vi "CODMn流程质控自动启动.vi"(0 "参数":T1={"是否启用仪器"=FALSE, "CODMn"={"启动测量模式"={"测量模式"=enum."水样测量"}, "确定按钮"=TRUE}, "启动模块"={"氨氮"=FALSE, "总磷"=FALSE, "总氮"=FALSE, "COD"=FALSE}, "常规启动"=FALSE, "直接启动"=FALSE}, 1 "CODMn量程切换":enum32{"H", "L", "AUTO"}(ring)=enum."AUTO") -> ()   [LabVIEW 2016, in "质控单元.lvlib"]
uses:
  PLC/PLC.lvlib
panel:
  out "枚举 2":enum16{"初始化", "采配水启动", "等待", "配水", "排水", "结束"}(ring)
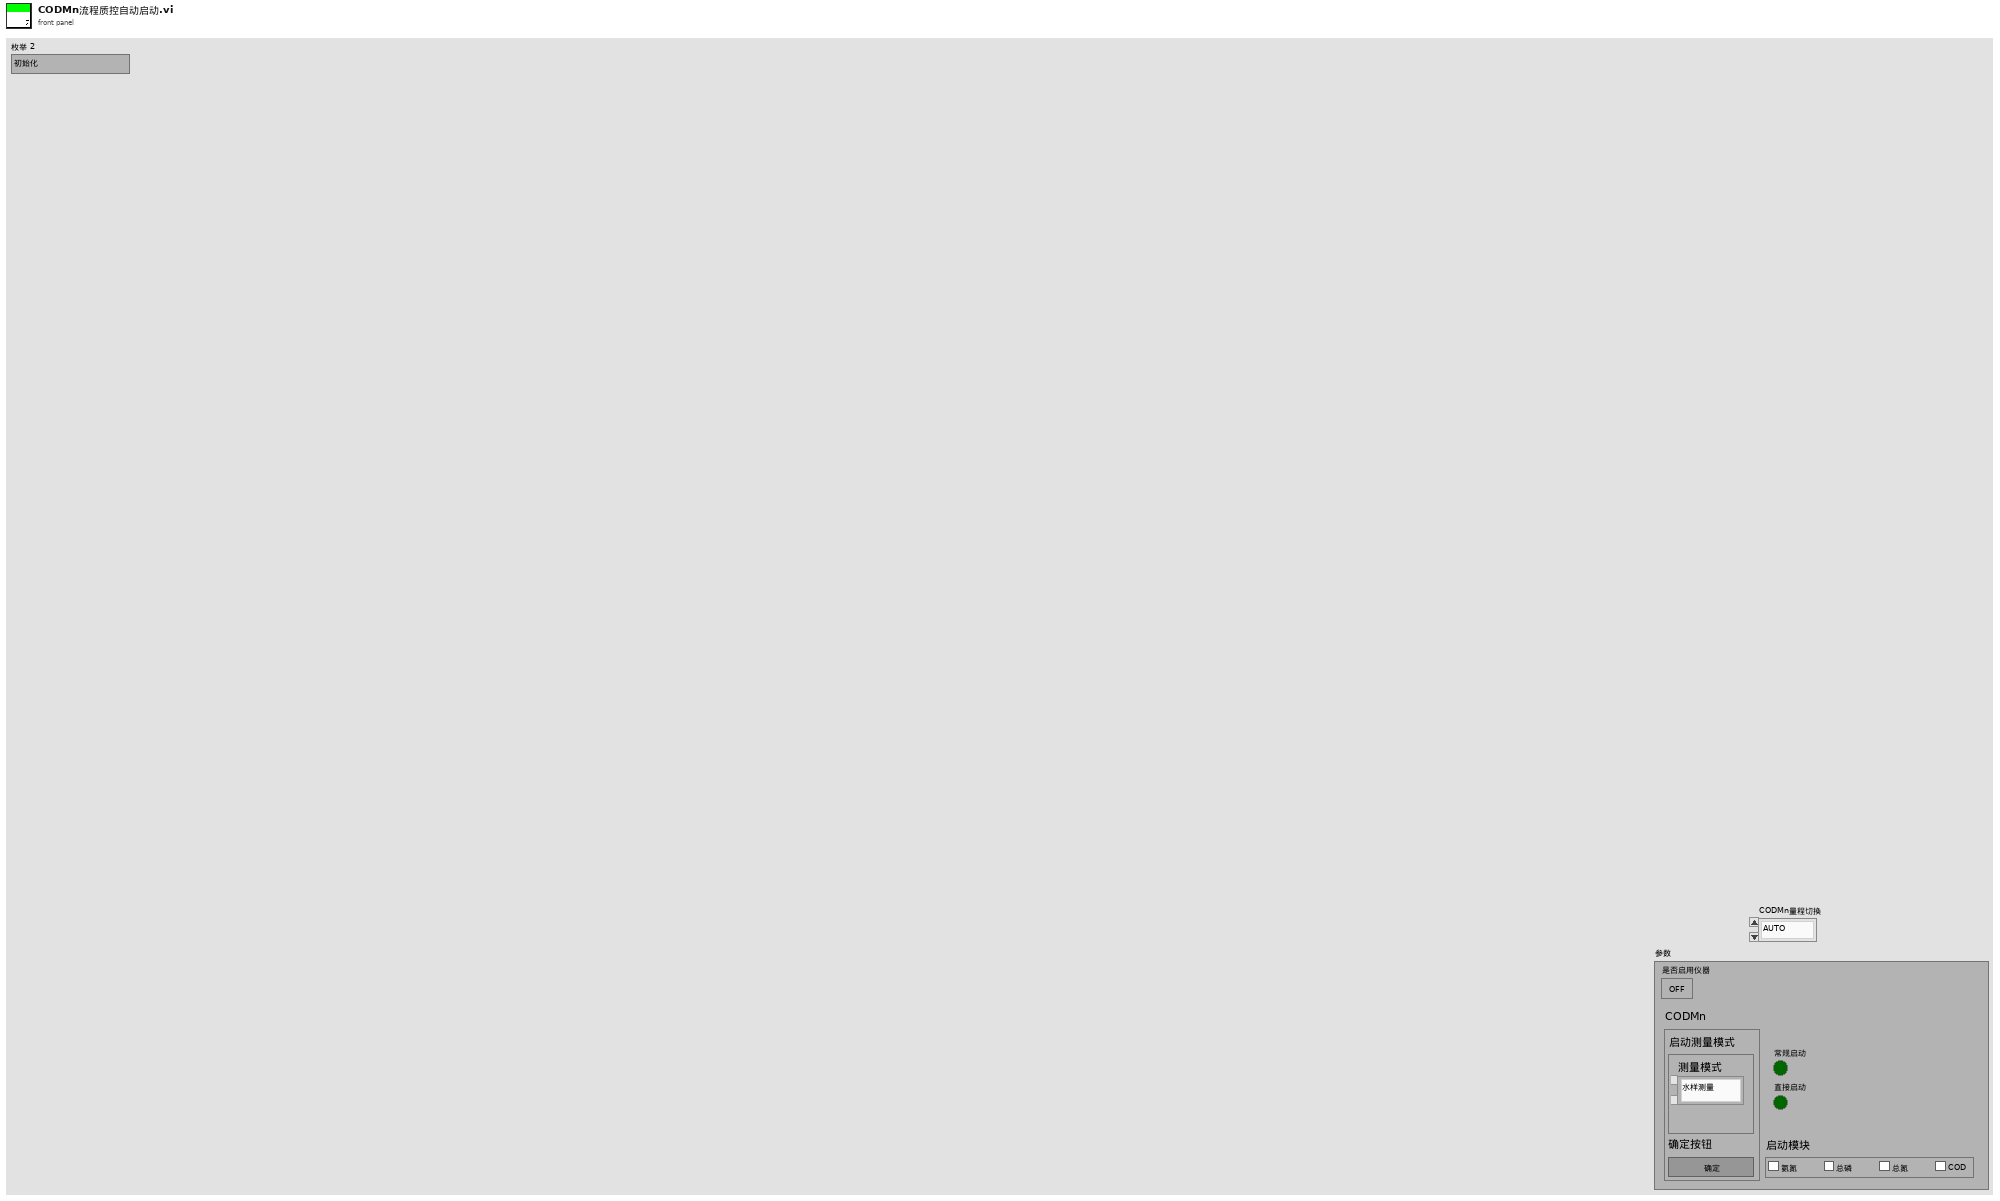
[diagram p1: front panel]
types:
  T1 = cluster{"是否启用仪器":bool, "CODMn":cluster{"启动测量模式":cluster{"测量模式":enum16{"水样测量", "标样核查", "加标回收", "平行样", "校零", "校标"}}, "确定按钮":bool}, "启动模块":cluster{"氨氮":bool, "总磷":bool, "总氮":bool, "COD":bool}, "常规启动":bool, "直接启动":bool}
  T2 = cluster{"R0":i16, "R1":i16, "R2":i16, "R3":i16, "R4":i16, "R5":i16, "R6":i16, "R7":i16, "R8":i16, "R9":i16, "R10":i16, "R11":i16, "R12":i16, "R13":i16, "R14":i16, "R15":i16, "R16":i16, "R17":i16, "R18":i16, "R19":i16, "R20":i16, "R21":i16, "R22":i16, "R23":i16, "R24":i16, "R25":i16, "R26":i16, "R27":i16, "R28":i16, "R29":i16, "R30":i16, "R31":i16, "R32":i16, "R33":i16, "R34":i16, "R35":i16, "R36":i16, "R37":i16, "R38":i16, "R39":i16, "R40":i16, "R41":i16, "R42":i16, "R43":i16, "R44":i16, "R45":i16, "R46":i16, "R47":i16, "R48":i16, "R49":i16, "R50":i16, "R51":i16, "R52":i16, "R53":i16, "R54":i16, "R55":i16, "R56":i16}
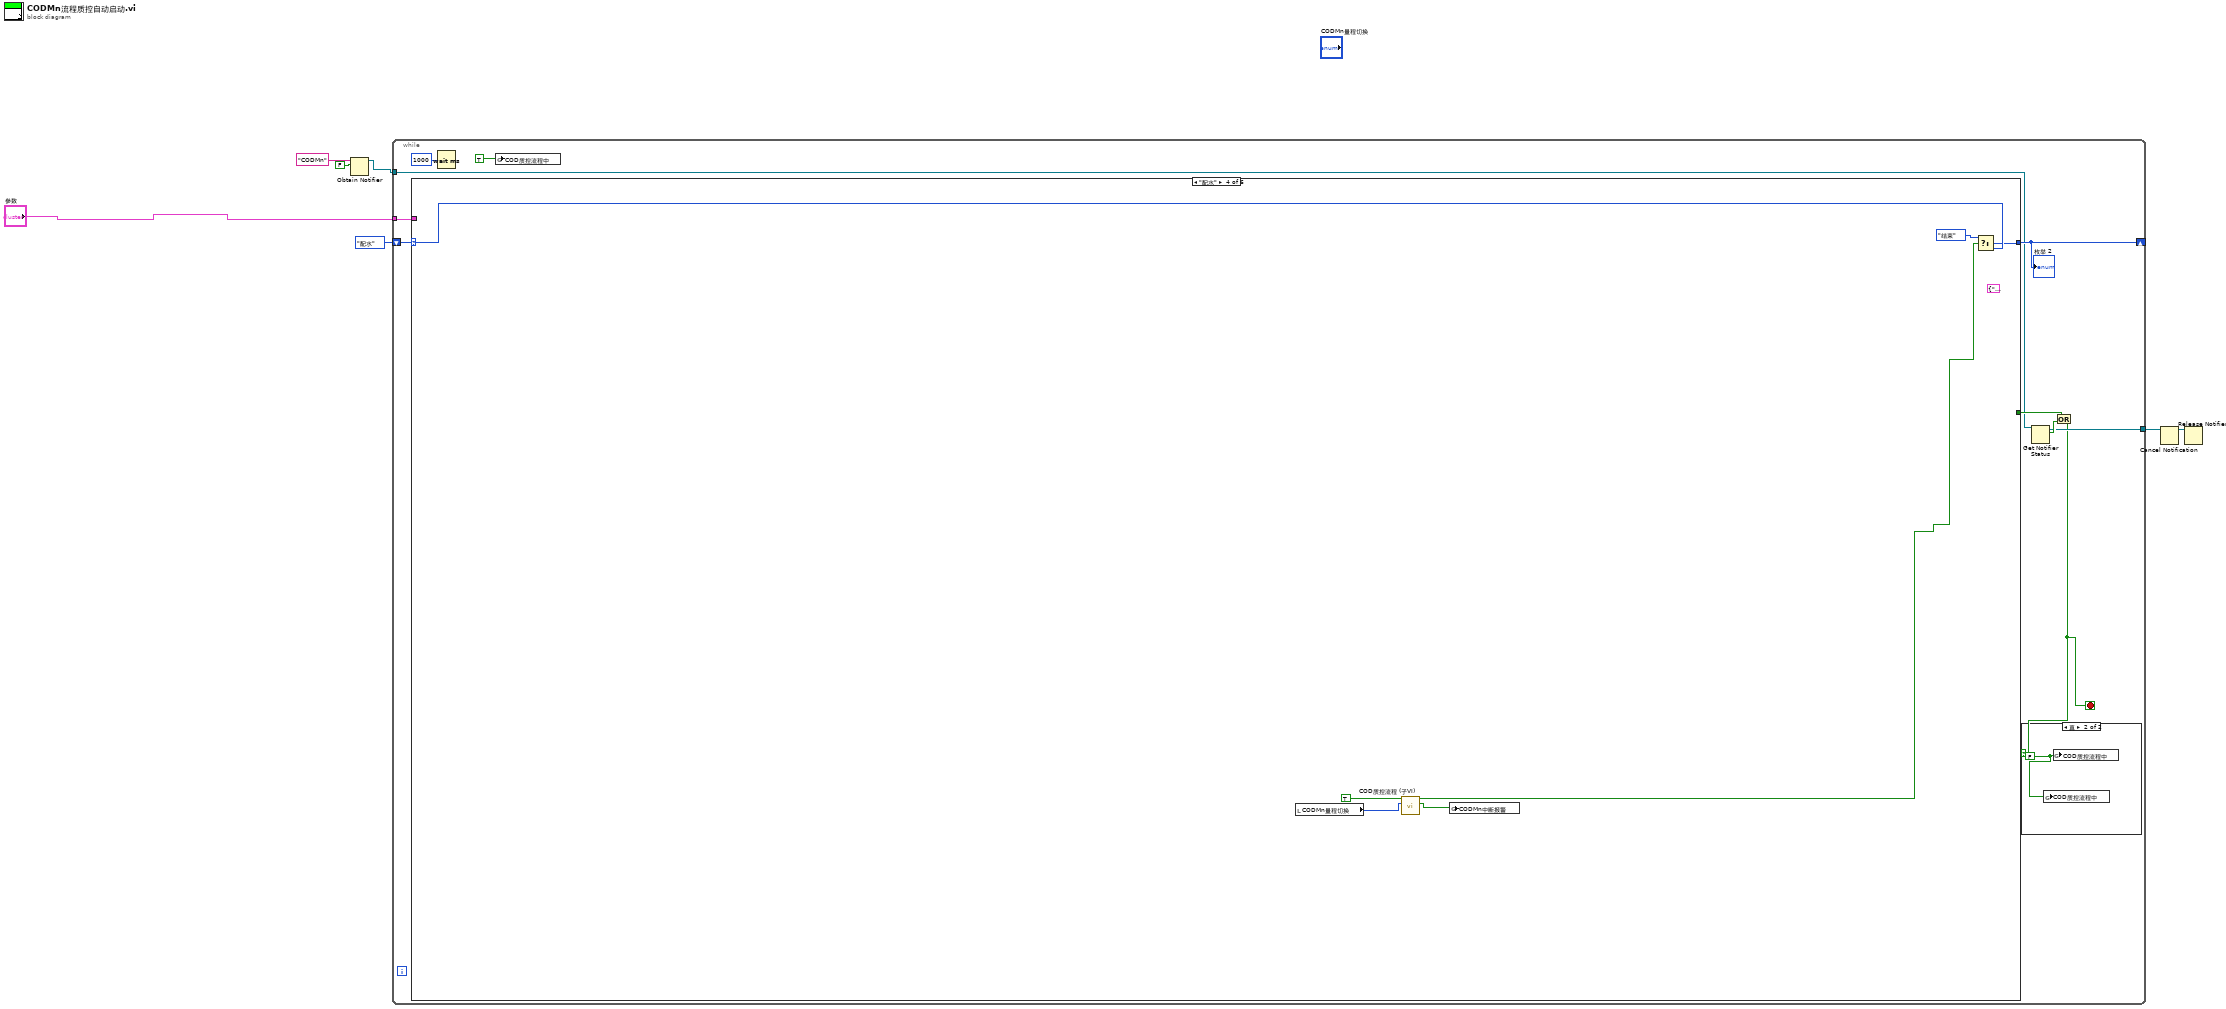
[diagram p0: block diagram]
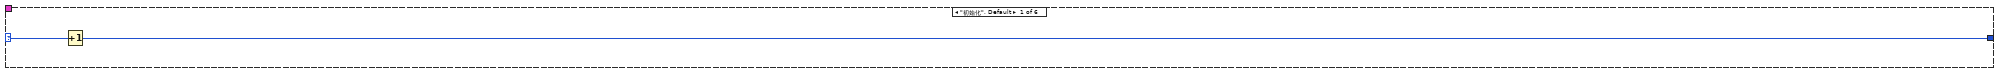
[diagram p3: hidden frame]
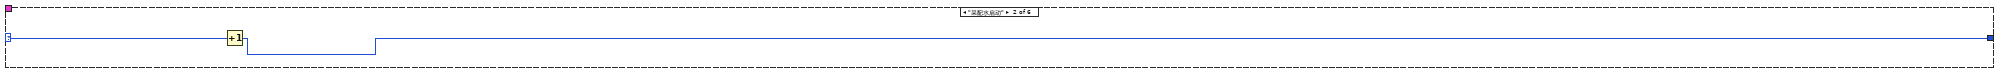
[diagram p4: hidden frame]
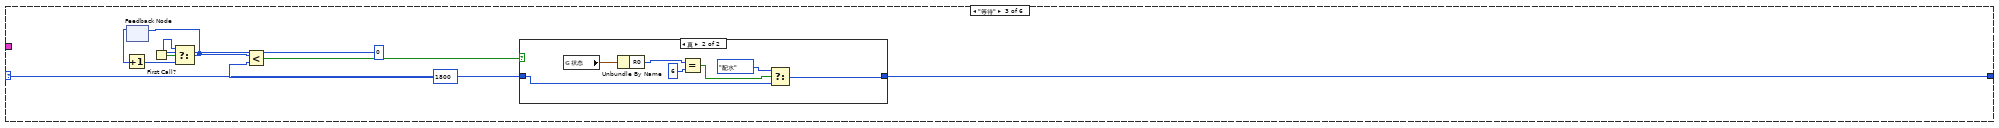
[diagram p5: hidden frame]
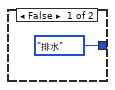
[diagram p6: hidden frame]
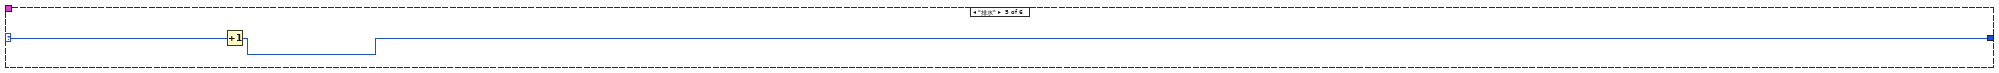
[diagram p7: hidden frame]
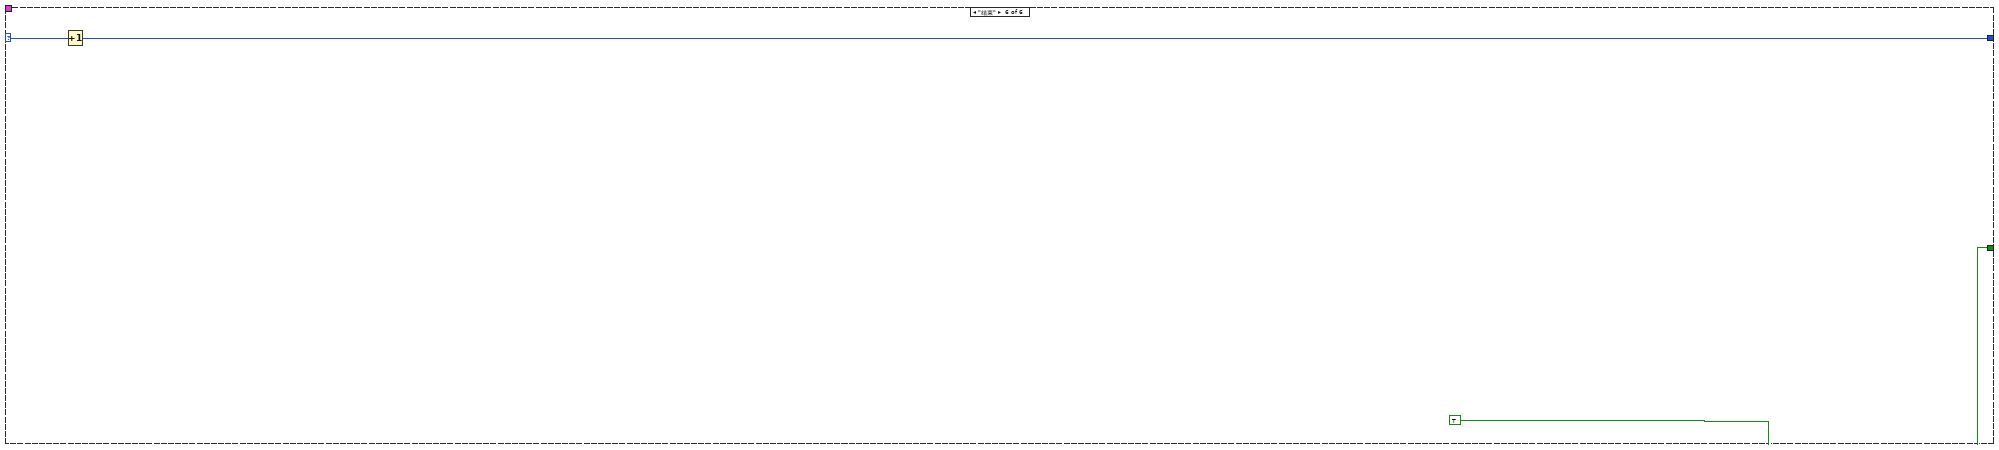
[diagram p8: hidden frame]
diagram:
  n1 = Obtain Notifier(name (unnamed)="CODMn" ("名称（未命名）"), notification data type=FALSE) -> (notifier out=w3:refnum<notifier>)  [unwired: 2 in, 2 out]
  n2 = while {
    shift-right: [w16] -> _
    shift-left: enum16{"初始化", "采配水启动", "等待", "配水", "排水", "结束"}."配水" ("枚举") -> [w17]
    tunnel: "参数" -> [w14]
    tunnel: w3 -> [w11]
    tunnel: [w10] -> w1
    stop <- w8 stop-if-true
    n3 = case shown="\"配水\"" w17 {
      selector: w17 -> [w20 w22 w29 w45 w48 w51]
      tunnel: [w19 w21 w28 w44 w47 w50] -> w16
      tunnel: [_ _ _ _ _ TRUE] -> w13
      tunnel: w14 -> [_ _ _ _ _ _]
      frame "初始化", Default {
        n4 = Increment(x=w20) -> (x+1=w19:enum16{"初始化", "采配水启动", "等待", "配水", "排水", "结束"})
      }
      frame "采配水启动" {
        n5 = Increment(x=w22) -> (x+1=w21:enum16{"初始化", "采配水启动", "等待", "配水", "排水", "结束"})
      }
      frame "等待" {
        n6 = feedback #1() -> (w25:i32)  [unwired: 1 in]
        n7 = Increment(x=w25) -> (x+1=w24:i32)
        n8 = First Call?() -> (First Call?: T/F=w26:bool)
        n9 = Select(t=0, s=w26, f=w24) -> (s? t:f=w23:i32)
        n10 = feedback-in #1(w23) -> ()
        n11 = Less?(x=w23, y=1800) -> (x < y?=w30:bool)
        n12 = case shown="真" w30 {
          tunnel: w29 -> [_ w34]
          tunnel: [enum16{"初始化", "采配水启动", "等待", "配水", "排水", "结束"}."排水" ("枚举") w33] -> w28
          frame False {
          }
          frame True {
            n13 = global read "采配水全局变量.vi" "状态"() -> (w39:T2)
            n14 = Unbundle By Name(w39) -> ("R0"=w38:i16)
            n15 = Equal?(x=w38, y=i16 6) -> (x = y?=w36:bool)
            n16 = Select(t=enum16{"初始化", "采配水启动", "等待", "配水", "排水", "结束"}."配水" ("枚举"), s=w36, f=w34) -> (s? t:f=w33:enum16{"初始化", "采配水启动", "等待", "配水", "排水", "结束"})
          }
        }
      }
      frame "配水" {
        (unwired) cluster{"命令":string, "data":variant} {"命令"="启动", "data"=variant(cluster{"站号":u16, "控制命令输出":u16[]} {"站号"=1, "控制命令输出"=[256, 0]})} ("元素")
        n17 = local read "CODMn量程切换"() -> (w42:enum32{"H", "L", "AUTO"})
        n18 = call "COD质控流程 (子VI).vi"("CODMn量程切换"=w42, "COD"=TRUE) -> ("CODMn中断报警"=w40:bool, "布尔"=w41:bool)  [unwired: 8 in]
        n19 = global write "质控中断报警全局.vi" "CODMn中断报警"(w40) -> ()
        n20 = Select(t=enum16{"初始化", "采配水启动", "等待", "配水", "排水", "结束"}."结束" ("枚举"), s=w41, f=w45) -> (s? t:f=w44:enum16{"初始化", "采配水启动", "等待", "配水", "排水", "结束"})
      }
      frame "排水" {
        n21 = Increment(x=w48) -> (x+1=w47:enum16{"初始化", "采配水启动", "等待", "配水", "排水", "结束"})
      }
      frame "结束" {
        n22 = Increment(x=w51) -> (x+1=w50:enum16{"初始化", "采配水启动", "等待", "配水", "排水", "结束"})
      }
    }
    "枚举 2" <- w16
    n23 = Wait (ms)(milliseconds to wait=u32 1000 ("等待时间（毫秒）")) -> ()  [unwired: 1 out]
    n24 = global write "质控测完标志全局 1.vi" "COD质控流程中"(TRUE ("氨氮质控流程中")) -> ()
    n25 = Get Notifier Status(notifier=w11) -> (notifier out=w10:refnum<notifier>, current notification=w12:bool)  [unwired: 1 in, 3 out]
    n26 = Or(x=w13, y=w12) -> (x .or. y?=w8:bool)
    n27 = case shown="真" w8 {
      frame False {
      }
      frame True {
        w18 = FALSE ("氨氮质控流程中")
        n28 = global write "质控测完标志全局 1.vi" "COD质控流程中"(w18) -> ()
        n29 = global write "质控测完标志全局 1.vi" "COD质控流程中"(w18) -> ()
      }
    }
  }
  n30 = Cancel Notification(0:w1) -> (8:w2:refnum<notifier>)  [unwired: 1 in, 2 out]
  n31 = Release Notifier(notifier=w2) -> ()  [unwired: 2 in, 3 out]
